vi "Forcade_Size_Set.vi"(8 "error in (no error)":errorcluster caption="错误输入（无错误）", 10 "Draw Area Size":T1, 11 "Picture_Class 输入":refnum<class "Picture_Class.lvclass"> caption="DNL_LabVIEW Object in") -> (0 "error out":errorcluster caption="错误输出", 3 "Picture_Class 输出":refnum<class "Picture_Class.lvclass"> caption="DNL_LabVIEW Object out")   [LabVIEW 2013, in "Picture_Class.lvclass"]
uses:
  Picture_Class.lvclass
  <vilib>/Utility/miscctls.llb/LVBoundsTypeDef.ctl
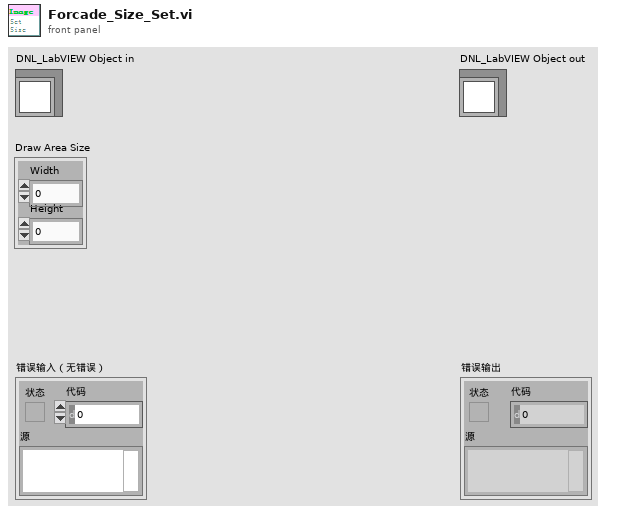
[diagram p1: front panel]
types:
  T1 = typedef "LVBoundsTypeDef.ctl" = cluster{"Width":u32, "Height":u32}
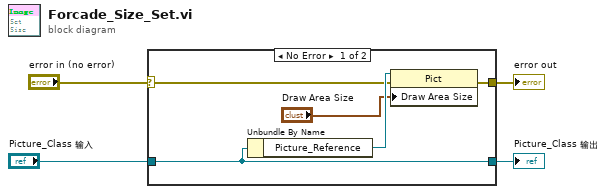
[diagram p0: block diagram]
diagram:
  n1 = case shown="No Error" "error in (no error)" {
    selector: "error in (no error)" -> [w6 w11]
    tunnel: [w8 w11] -> w3
    tunnel: [w9 w10] -> w1
    tunnel: "Picture_Class 输入" -> [w9 w10]
    frame No Error {
      n2 = Unbundle By Name(w9) -> ("Picture_Reference"=w7:refnum<vi>)
      n3 = property class="Pict"(reference=w7, error in=w6, "Draw Area Size"="Draw Area Size") -> (error out=w8:errorcluster)  [unwired: 1 out]
    }
    frame Error {
    }
  }
  "error out" <- w3
  "Picture_Class 输出" <- w1
